vi "Sync Config from Instr.vi"(8 "error in (no error)":errorcluster, 11 "Cryo-Con Driver in":refnum<class "Cryo-Con Driver.lvclass">) -> (0 "error out":errorcluster, 2 "Variant":variant, 3 "Cryo-Con Driver out":refnum<class "Cryo-Con Driver.lvclass">)   [LabVIEW 2021, in "Cryo-Con Driver.lvclass"]
uses:
  Cryo-Con Driver.lvclass
  C:/GitHub/NHMFL_Core/Libraries/Instruments/VISA Instrument/VISA Instrument.lvclass
  C:/GitHub/NHMFL_Core/Libraries/Instruments/Temperature Controller Driver/Temperature Controller Driver.lvclass
  VISA Instrument/VISA Instrument.lvclass/VISA Instrument.ctl
  VISA Instrument/Read VISA resource.vi
  VISA Instrument/Write VISA resource.vi
  Temperature Controller Driver/Read T controller configuration.vi
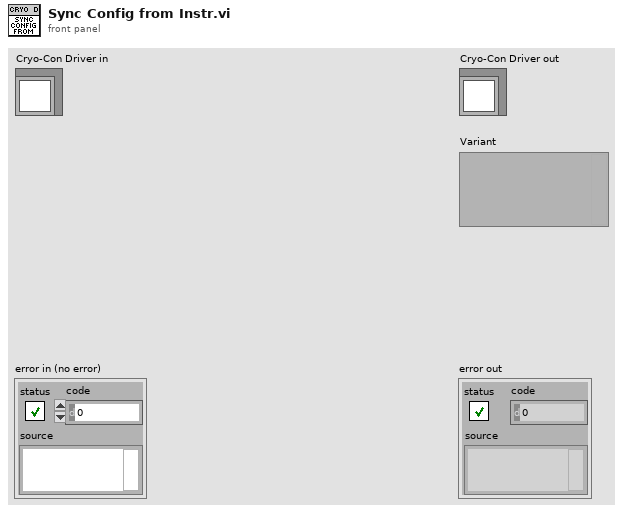
[diagram p1: front panel]
types:
  T1 = typedef "T controller configuration.ctl" = cluster{"Record Channels":string[], "Record raw signal":bool, "Set point":dbl, "Record heater":bool, "Ramp rate":dbl, "P":dbl, "I":dbl, "D":dbl, "Control":T2, "P manual":dbl, "Output #":i32}
  T2 = typedef "Control Mode.ctl" = enum16{"Off", "PID", "Ramp", "Manual", "Table"}
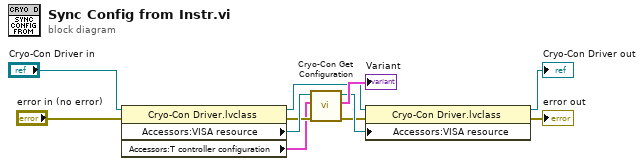
[diagram p0: block diagram]
diagram:
  n1 = property class="Cryo-Con Driver.lvclass"(reference="Cryo-Con Driver in", error in="error in (no error)") -> (reference out=w7:refnum<class "Cryo-Con Driver.lvclass">, error out=w3:errorcluster, "Accessors:VISA resource"=w9:refnum<visa-resource-name>, "Accessors:T controller configuration"=w1:T1)
  n2 = call "Cryo-Con Get Configuration.vi"("Error In"=w3, "Config"=w1, "VISA resource name"=w9) -> ("Error Out"=w2:errorcluster, "Config out"=→"Variant":T1, "VISA resource name out"=w4:refnum<visa-resource-name>)  [unwired: 6 in]
  n3 = property class="Cryo-Con Driver.lvclass"(reference=w7, error in=w2, "Accessors:VISA resource"=w4) -> (reference out=→"Cryo-Con Driver out":refnum<class "Cryo-Con Driver.lvclass">, error out=→"error out":errorcluster)
